vi "Main.vi"() -> ()   [LabVIEW 2017]
doc: "This Continuous Measurement sample project is based on the Queued Message Handler template.\n\nThe Event Handling Loop generates messages based on user interface actions.\n\nThe Message Handling Loop processes messages generated by the Event Handling Loop, or by other messages. There are also Acquisition and Logging message handling loop subVIs, and a chart updating loop."
uses:
  Settings/Settings.ctl
  Acquisition/Hardware Configuration.ctl
  Acquisition/Signal Type.ctl
  Logging/Logging Configuration.ctl
  controls/UI Data.ctl
  controls/UI State.ctl
  support/Message Queue/Enqueue Message (Single).vi
  support/Message Queue/Enqueue Message (Array).vi
  <vilib>/Utility/error.llb/Error Cluster From Error Code.vi
  <vilib>/ErrorRing/Error Ring.xnode
  Acquisition/Acquisition.lvlib
  Logging/Logging.lvlib
  Settings/Settings.lvlib
  support/User Event - Stop/User Event - Stop.lvlib
  support/Message Queue/Message Queue.lvlib
  Settings/Settings Dialog.vi
panel:
  out "Time running":timestamp format="%<%H:%M:%S%1u>T"
  in  "Zero run?":bool
  in  "Start wavemaker":bool
  in  "Preview wave file":bool
  out "Data wave file":waveform(dbl)[](graph)
  in  "Initialize wave maker":bool
  in  "Location wave file":path
  in  "Configure channels":bool
  in  "Exit":bool
  out "Status":string
  in  "Settings":bool
  in  "Stop":bool
  in  "Start":bool
  out "ChannelNames":T1
  out "Offline storage?":bool
  out "Path to offsite data storage":path
  in  "Close and start writing time interval [min]":dbl
  out "Project  code":string
  in  "Zero run testing time [s]":dbl
  in  "Testing time [m]":dbl
  out "Data":waveform(dbl)[](graph)
  # "Flume tank data logging and wave making"
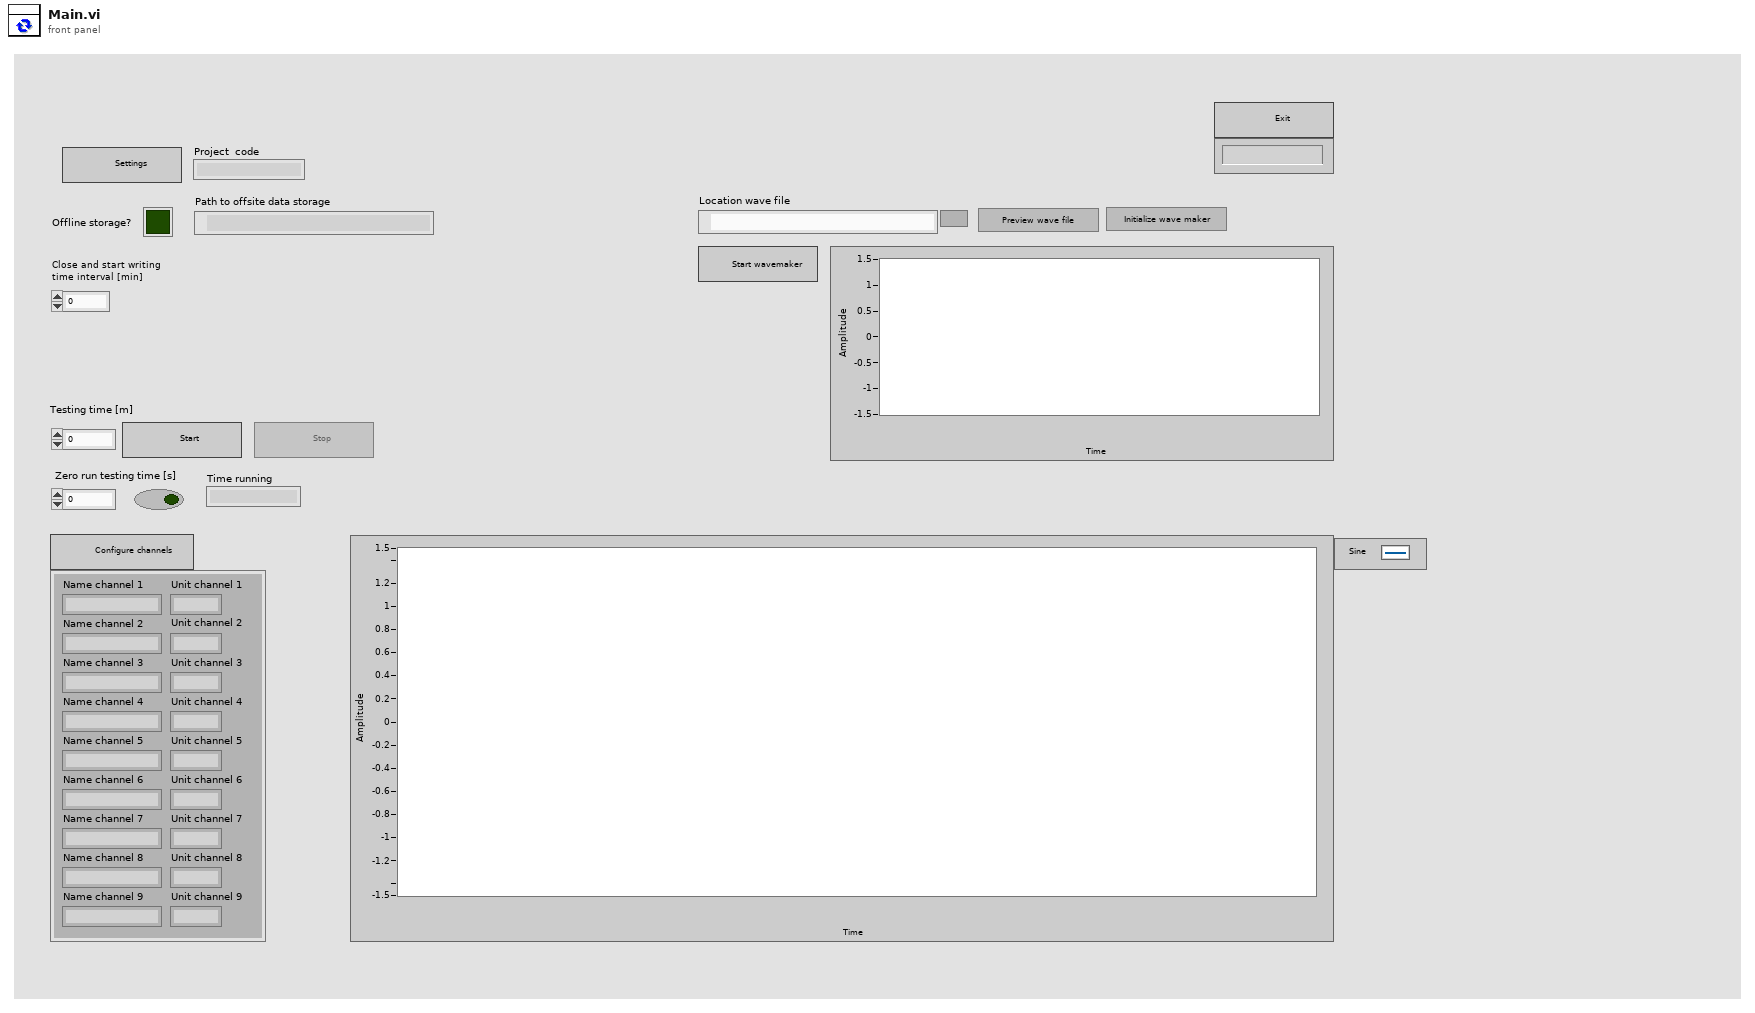
[diagram p1: front panel]
types:
  T1 = cluster{"Name channel 1":string, "Name channel 2":string, "Name channel 3":string, "Name channel 4":string, "Name channel 5":string, "Name channel 6":string, "Name channel 7":string, "Name channel 8":string, "Name channel 9":string, "Unit channel 1":string, "Unit channel 2":string, "Unit channel 3":string, "Unit channel 4":string, "Unit channel 5":string, "Unit channel 6":string, "Unit channel 7":string, "Unit channel 8":string, "Unit channel 9":string}
  T2 = typedef "UI State.ctl" = enum16{"Idle", "Acquiring and Logging", "Waiting for Exit", "Waiting for Exit (Acq Stopped)", "Waiting for Exit (Log Stopped)", "Waiting for Stop", "Waiting for Stop (Acq Stopped)", "Waiting for Stop (Log Stopped)"}
  T3 = typedef "UI Data.ctl" = cluster{"Start Ref":refnum<vi>, "Stop Ref":refnum<vi>, "Settings Ref":refnum<vi>, "Exit Ref":refnum<vi>, "Status Ref":refnum<vi>, "Data Ref":refnum<vi>, "Start wavemaker ref":refnum<vi>, "Preview wave file ref":refnum<vi>, "Config channels ref":refnum<vi>, "Wave preview ref":refnum<vi>}
  T4 = typedef "Settings.lvlib/Settings.ctl" = cluster{"Hardware Configuration":T5, "Logging Configuration":T7, "Project  code":string, "Offline storage?":bool, "Path to offsite data storage":path}
  T5 = typedef "Acquisition.lvlib/Hardware Configuration.ctl" = cluster{"HW Refnum <Replace Me>":string, "Signal Type <Replace Me>":T6}
  T6 = typedef "Acquisition.lvlib/Signal Type.ctl" = enum16{"Sine Wave", "Square with Noise"}
  T7 = typedef "Logging.lvlib/Logging Configuration.ctl" = cluster{"Log File Base Path":path, "TDMS File Reference":refnum<k34>}
  T8 = typedef "Message Queue.lvlib/All Message Queues.ctl" = cluster{"UI":refnum<queue>, "Acquisition":refnum<queue>, "Logging":refnum<queue>}
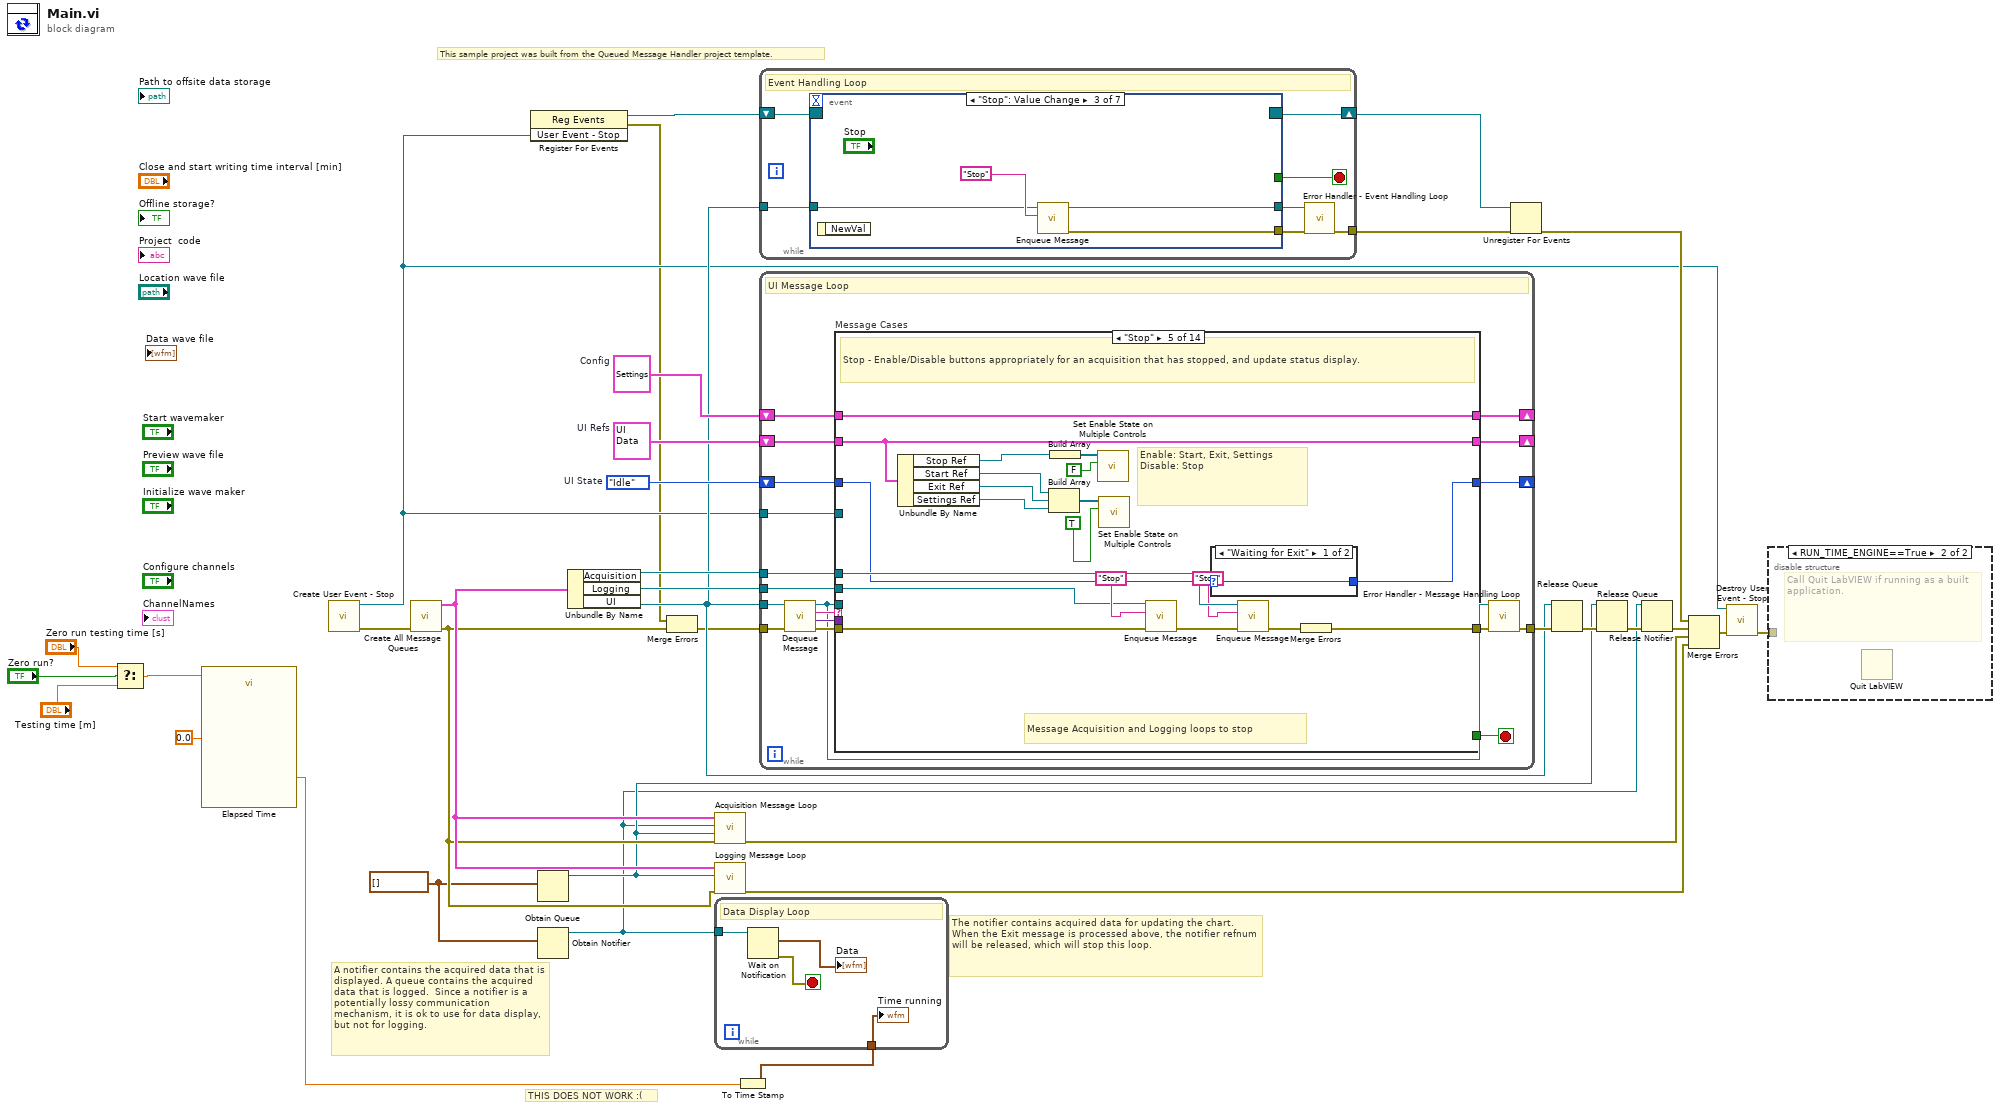
[diagram p0: block diagram]
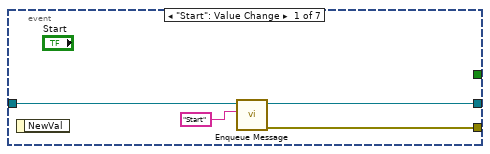
[diagram p3: hidden frame]
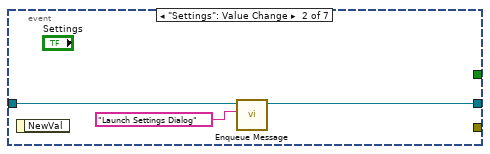
[diagram p4: hidden frame]
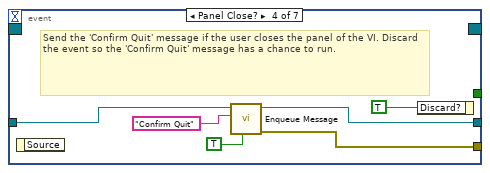
[diagram p5: hidden frame]
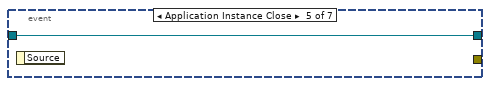
[diagram p6: hidden frame]
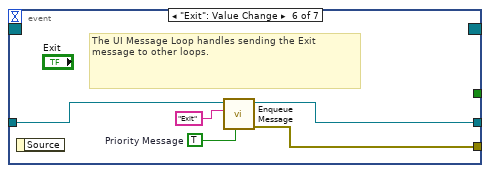
[diagram p7: hidden frame]
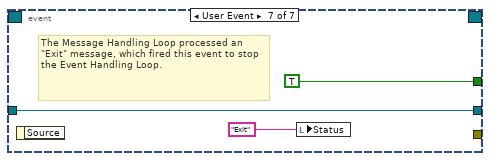
[diagram p8: hidden frame]
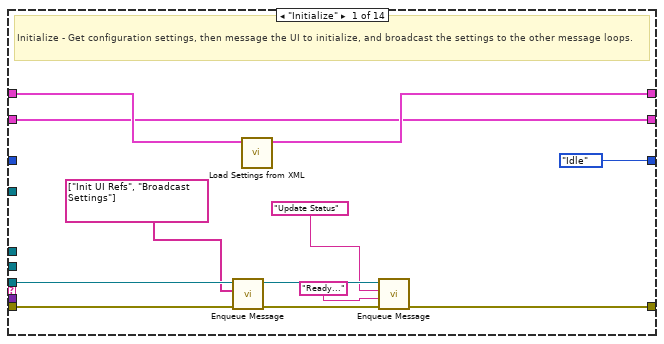
[diagram p9: hidden frame]
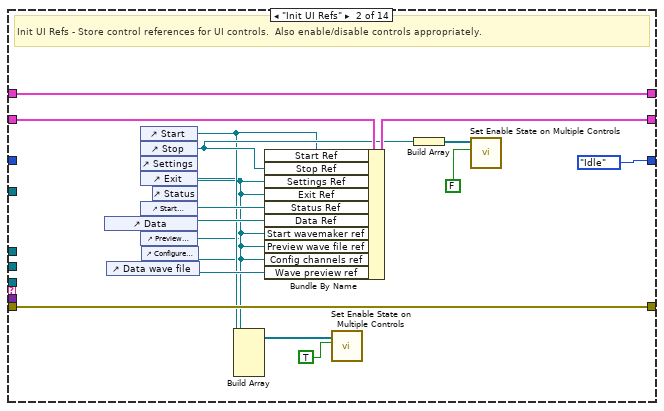
[diagram p10: hidden frame]
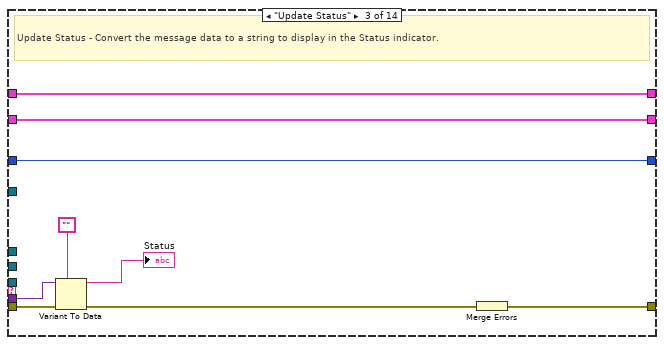
[diagram p11: hidden frame]
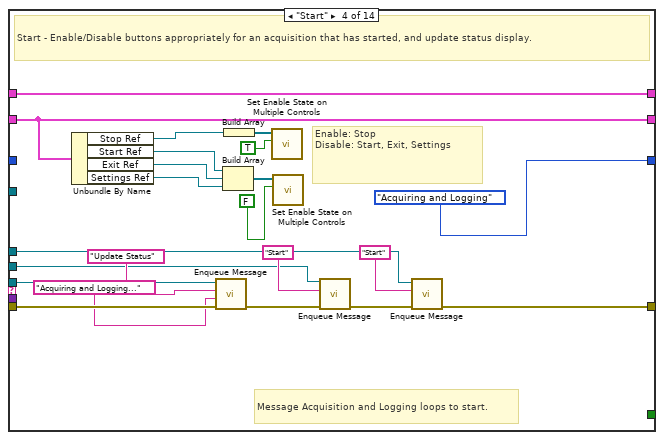
[diagram p12: hidden frame]
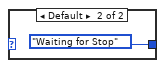
[diagram p13: hidden frame]
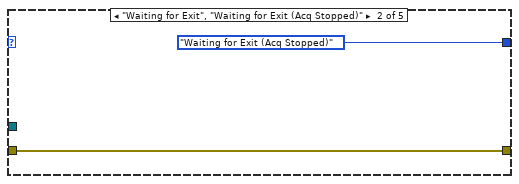
[diagram p15: hidden frame]
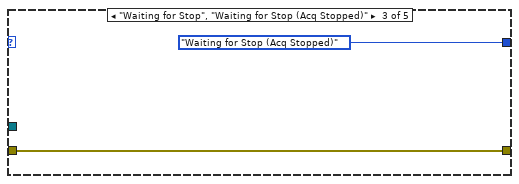
[diagram p16: hidden frame]
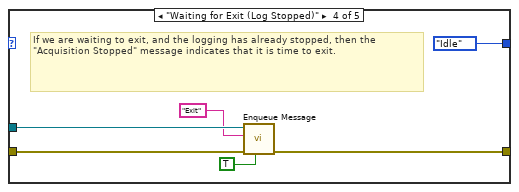
[diagram p17: hidden frame]
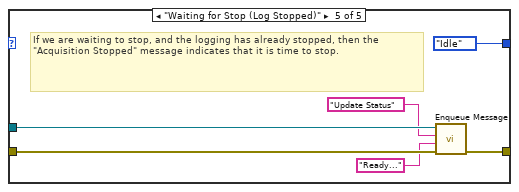
[diagram p18: hidden frame]
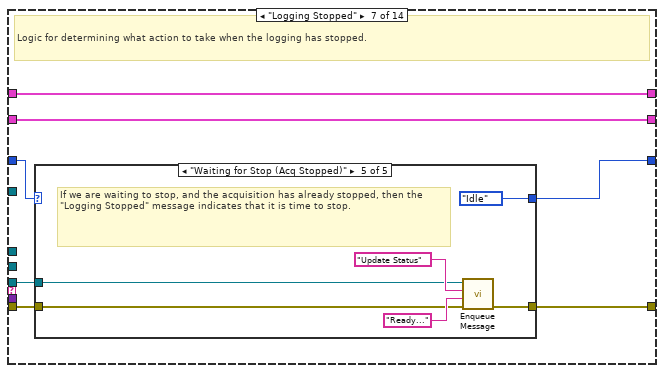
[diagram p19: hidden frame]
diagram:
  w21 = UI_State."Idle"  # UI State
  w12 = waveform(dbl)[] []
  w24 = T3 {"Start Ref"=refnum, "Stop Ref"=refnum, "Settings Ref"=refnum, "Exit Ref"=refnum, "Status Ref"=refnum, "Data Ref"=refnum, "Start wavemaker ref"=refnum, "Preview wave file ref"=refnum, "Config channels ref"=refnum, "Wave preview ref"=refnum}  # UI Refs
  w27 = T4 {"Hardware Configuration"={"HW Refnum <Replace Me>"="", "Signal Type <Replace Me>"=enum."Sine Wave"}, "Logging Configuration"={"Log File Base Path"=path "", "TDMS File Reference"=refnum}, "Project  code"="", "Offline storage?"=FALSE, "Path to offsite data storage"=path ""}  # Config
  # "THIS DOES NOT WORK :("
  # "This sample project was built from the Queued Message Handler project template."
  # "A notifier contains the acquired data that is displayed. A queue contains the acquired data that is logged.  Since a notifier is a potentially lossy communication mechanism, it is ok to use for data display, but not for logging."
  # "The notifier contains acquired data for updating the chart. When the Exit message is processed above, the notifier refnum will be released, which will stop this loop."
  n1 = Select(t="Zero run testing time [s]", s="Zero run?", f="Testing time [m]") -> (s? t:f=w4:dbl)
  n2 = call "Elapsed Time"("Time Target (s)"=w4, "Set Start Time (s)"=0.0) -> ("Elapsed Time (s)"=w1:dbl)  [unwired: 10 in, 7 out]
  n3 = call "Create User Event - Stop.vi"() -> ("error out"=w31:errorcluster, "User Event - Stop"=w10:refnum<user-event>)  [unwired: 10 in]
  n4 = call "Create All Message Queues.vi"("error in (no error)"=w31) -> ("error out"=w28:errorcluster, "Message Queues out"=w30:T8)  [unwired: 9 in]
  n5 = register-events(w10) -> (reference out=w11:refnum<event-registration>, error out=w8:errorcluster)  [unwired: 2 in]
  n6 = Obtain Queue(element data type=w12) -> (queue out=w14:refnum<queue>)  [unwired: 4 in, 2 out]
  n7 = Obtain Notifier(notification data type=w12) -> (notifier out=w13:refnum<notifier>)  [unwired: 3 in, 2 out]
  n8 = Unbundle By Name(w30) -> ("Acquisition"=w23:refnum<queue>, "Logging"=w22:refnum<queue>, "UI"=w19:refnum<queue>)
  n9 = Merge Errors(w8, w28) -> (w9:errorcluster)
  n10 = call "Acquisition Message Loop.vi"("error in (no error)"=w28, "Data Queue"=w14, "Data Notifier"=w13, "Message Queues"=w30) -> ("error out"=w32:errorcluster)  [unwired: 7 in]
  n11 = call "Logging Message Loop.vi"("error in (no error)"=w28, "Data Queue"=w14, "Message Queues"=w30) -> ("error out"=w29:errorcluster)  [unwired: 8 in]
  n12 = To Time Stamp(1:w1) -> (0:w2:timestamp)
  n13 = while "Data Display Loop" {
    tunnel: w13 -> [w38]
    tunnel: w2 -> [w35]
    stop <- w36 stop-if-true
    # "Data Display Loop"
    n14 = Wait on Notification(notifier=w38) -> (notification=→"Data":waveform(dbl)[], error out=w36:errorcluster)  [unwired: 3 in, 2 out]
    "Time running" <- w35
  }
  n15 = while {
    tunnel: w19 -> [w44]
    tunnel: [w41] -> w33
    shift-right: [w43] -> w25
    shift-left: w11 -> [w45]
    stop <- w42 stop-if-true
    # "Event Handling Loop"
    n16 = event shown="[2] \"Stop\": Value Change" {
      selector: w45 -> [_ _ _ _ _ _ _]
      dyn-events: [_ _ _ _ _ _ _] -> w43
      timeout: _ -> [_ _ _ _ _ _ _]
      tunnel: [_ _ _ _ _ _ TRUE ("Discard?")] -> w42
      tunnel: w44 -> [w49 w51 w55 w60 w63 w65 w69]
      tunnel: [w47 _ w54 w58 _ w68 _] -> w40
      tunnel: [w46 w50 w53 w59 w63 w64 w69] -> w39
      event "Start": Value Change {
        n17 = event-data() -> ()  [unwired: 1 in, 1 out]
        n18 = call-poly "Enqueue Message.vi"("Message"="Start", "Message Queue"=w49) -> ("error out"=w47:errorcluster, "dup Message Queue"=w46:refnum<queue>)  [unwired: 8 in]
      }
      event "Settings": Value Change {
        n19 = event-data() -> ()  [unwired: 1 in, 1 out]
        n20 = call-poly "Enqueue Message.vi"("Message"="Launch Settings Dialog", "Message Queue"=w51) -> ("dup Message Queue"=w50:refnum<queue>)  [unwired: 8 in, 1 out]
      }
      event "Stop": Value Change {
        n21 = event-data() -> ()  [unwired: 1 in, 1 out]
        n22 = call-poly "Enqueue Message.vi"("Message"="Stop", "Message Queue"=w55) -> ("error out"=w54:errorcluster, "dup Message Queue"=w53:refnum<queue>)  [unwired: 8 in]
      }
      event Panel Close? {
        # "Send the 'Confirm Quit' message if the user closes the panel of the VI. Discard the event so the 'Confirm Quit' message has a chance to run."
        n23 = event-data() -> ()  [unwired: 1 in, 1 out]
        n24 = call-poly "Enqueue Message.vi"("Priority Message? (F)"=TRUE, "Message"="Confirm Quit", "Message Queue"=w60) -> ("error out"=w58:errorcluster, "dup Message Queue"=w59:refnum<queue>)  [unwired: 7 in]
        n25 = event-data("Discard?"=TRUE) -> ()  [unwired: 1 in, 1 out]
      }
      event Application Instance Close {
        n26 = event-data() -> ()  [unwired: 1 in, 1 out]
      }
      event "Exit": Value Change {
        w66 = TRUE  # Priority Message
        # "The UI Message Loop handles sending the Exit message to other loops."
        n27 = event-data() -> ()  [unwired: 1 in, 1 out]
        n28 = call-poly "Enqueue Message.vi"("Priority Message? (F)"=w66, "Message"="Exit", "Message Queue"=w65) -> ("error out"=w68:errorcluster, "dup Message Queue"=w64:refnum<queue>)  [unwired: 7 in]
      }
      event User Event {
        # "The Message Handling Loop processed an \"Exit\" message, which fired this event to stop the Event Handling Loop."
        n29 = event-data() -> ()  [unwired: 1 in, 1 out]
        n30 = local write "Status"("Exit" ("Exit String")) -> ()
      }
    }
    n31 = call "Error Handler - Event Handling Loop.vi"("error in (no error)"=w40, "Message Queue"=w39) -> ("dup error in"=w41:errorcluster)  [unwired: 8 in, 1 out]
  }
  n32 = while {
    tunnel: w19 -> [w83]
    tunnel: w10 -> [w88]
    shift-right: [w82] -> _
    shift-left: w27 -> [w81]
    shift-right: [w79] -> _
    shift-left: w24 -> [w80]
    tunnel: w23 -> [w78]
    tunnel: w22 -> [w77]
    shift-right: [w72] -> _
    shift-left: w21 -> [w73]
    tunnel: w9 -> [w87]
    tunnel: [w76] -> w34
    stop <- w89 stop-if-true
    # "UI Message Loop"
    n33 = call "Dequeue Message.vi"("error in (no error)"=w87, "Message Queue"=w83) -> ("error out"=w86:errorcluster, "Message Data"=w84:variant, "Message"=w85:string, "dup Message Queue"=w74:refnum<queue>)  [unwired: 6 in]
    n34 = case "Message Cases" shown="\"Stop\"" w85 {
      selector: w85 -> [_ _ _ _ _ _ _ _ _ _ _ _ _ w315]
      tunnel: w74 -> [w93 _ _ w151 _ w176 w201 _ w247 _ w268 _ _ _]
      tunnel: w86 -> [w92 w120 w128 w150 w170 w177 w202 w237 w249 w256 w267 w296 w313 _]
      tunnel: [w97 w120 w129 w133 w171 w174 w199 w241 w242 w259 w266 w306 w312 w314] -> w75
      tunnel: [_ _ _ _ _ _ _ _ _ _ _ TRUE _ _] -> w89
      tunnel: w84 -> [_ _ w127 _ _ _ _ _ _ w260 _ w294 _ _]
      tunnel: w88 -> [_ _ _ _ _ _ _ _ _ _ _ w307 _ _]
      tunnel: [w100 w119 w123 w149 w169 w180 w205 w239 w246 w264 w271 w305 w311 w318] -> w82
      tunnel: w81 -> [w101 w119 w123 w149 w169 w180 w205 w239 w250 w264 w271 w305 w311 w318]
      tunnel: w80 -> [w94 w114 w122 w146 w168 w179 w204 w236 w244 w263 w270 w304 w310 w317]
      tunnel: [w94 w113 w122 w146 w168 w179 w204 w236 w244 w263 w270 w304 w310 w317] -> w79
      tunnel: w78 -> [_ _ _ w132 w155 _ _ w235 _ _ _ w303 _ _]
      tunnel: w77 -> [_ _ _ w135 w158 _ _ w224 _ _ _ w302 _ _]
      tunnel: w73 -> [_ _ w121 _ w152 w178 w203 w234 w243 w258 w269 _ w309 w316]
      tunnel: [UI_State."Idle" ("UI State") UI_State."Idle" ("UI State") w121 UI_State."Acquiring and Logging" ("UI State") w153 w175 w200 w234 w243 w258 w265 UI_State."Idle" ("UI State") w309 w316] -> w72
      frame "Initialize" {
        # "Initialize - Get configuration settings, then message the UI to initialize, and broadcast the settings to the other message loops."
        n35 = call-poly "Enqueue Message.vi"("error in (no error)"=w92, "Message Array"=string[] ["Init UI Refs", "Broadcast Settings"], "Message Queue"=w93) -> ("error out"=w99:errorcluster, "dup Message Queue"=w98:refnum<queue>)  [unwired: 7 in]
        n36 = call "Load Settings from XML.vi"("Settings in"=w101) -> ("Settings out"=w100:T4)  [unwired: 9 in, 1 out]
        n37 = call-poly "Enqueue Message.vi"("error in (no error)"=w99, "Message Data"="Ready..." ("Ready..."), "Message"="Update Status", "Message Queue"=w98) -> ("error out"=w97:errorcluster)  [unwired: 6 in, 1 out]
      }
      frame "Init UI Refs" {
        # "Init UI Refs - Store control references for UI controls.  Also enable/disable controls appropriately."
        n38 = control-ref of="Data"() -> (w110:refnum<vi>)
        n39 = control-ref of="Data wave file"() -> (w109:refnum<vi>)
        n40 = control-ref of="Start"() -> (w108:refnum<vi>)
        n41 = control-ref of="Stop"() -> (w112:refnum<vi>)
        n42 = control-ref of="Settings"() -> (w107:refnum<vi>)
        n43 = control-ref of="Exit"() -> (w106:refnum<vi>)
        n44 = control-ref of="Start wavemaker"() -> (w105:refnum<vi>)
        n45 = control-ref of="Preview wave file"() -> (w104:refnum<vi>)
        n46 = control-ref of="Configure channels"() -> (w103:refnum<vi>)
        n47 = control-ref of="Status"() -> (w111:refnum<vi>)
        n48 = Build Array(w108, w107, w106, w105, w104, w103) -> (w102:refnum<vi>[])
        n49 = Bundle By Name(cluster=w114, "Start Ref"=w108, "Stop Ref"=w112, "Settings Ref"=w107, "Exit Ref"=w106, "Status Ref"=w111, "Data Ref"=w110, "Start wavemaker ref"=w105, "Preview wave file ref"=w104, "Config channels ref"=w103, "Wave preview ref"=w109) -> (w113:T3)
        n50 = call "Set Enable State on Multiple Controls.vi"("Enable?"=TRUE, "Controls"=w102) -> ()  [unwired: 10 in]
        n51 = Build Array(w112) -> (w117:refnum<vi>[])
        n52 = call "Set Enable State on Multiple Controls.vi"("Enable?"=FALSE, "Controls"=w117) -> ()  [unwired: 10 in]
      }
      frame "Update Status" {
        # "Update Status - Convert the message data to a string to display in the Status indicator."
        n53 = Variant To Data(error in=w128, type="", Variant=w127) -> (data=→"Status":string, error out=w125:errorcluster)
        n54 = Merge Errors(w125) -> (w129:errorcluster)
      }
      frame "Start" {
        # "Message Acquisition and Logging loops to start."
        # "Enable: Stop\nDisable: Start, Exit, Settings"
        # "Start - Enable/Disable buttons appropriately for an acquisition that has started, and update status display."
        n55 = Unbundle By Name(w146) -> ("Stop Ref"=w141:refnum<vi>, "Start Ref"=w140:refnum<vi>, "Exit Ref"=w139:refnum<vi>, "Settings Ref"=w138:refnum<vi>)
        n56 = call-poly "Enqueue Message.vi"("error in (no error)"=w150, "Message Data"="Acquiring and Logging..." ("Acquiring and Logging..."), "Message"="Update Status", "Message Queue"=w151) -> ("error out"=w137:errorcluster)  [unwired: 6 in, 1 out]
        n57 = Build Array(w140, w139, w138) -> (w144:refnum<vi>[])
        n58 = Build Array(w141) -> (w143:refnum<vi>[])
        n59 = call "Set Enable State on Multiple Controls.vi"("Enable?"=TRUE, "Controls"=w143) -> ()  [unwired: 10 in]
        n60 = call "Set Enable State on Multiple Controls.vi"("Enable?"=FALSE, "Controls"=w144) -> ()  [unwired: 10 in]
        n61 = call-poly "Enqueue Message.vi"("error in (no error)"=w137, "Message"="Start", "Message Queue"=w135) -> ("error out"=w134:errorcluster)  [unwired: 7 in, 1 out]
        n62 = call-poly "Enqueue Message.vi"("error in (no error)"=w134, "Message"="Start", "Message Queue"=w132) -> ("error out"=w133:errorcluster)  [unwired: 7 in, 1 out]
      }
      frame "Stop" {
        # "Message Acquisition and Logging loops to stop"
        # "Enable: Start, Exit, Settings\nDisable: Stop"
        # "Stop - Enable/Disable buttons appropriately for an acquisition that has stopped, and update status display."
        n63 = Unbundle By Name(w168) -> ("Stop Ref"=w163:refnum<vi>, "Start Ref"=w162:refnum<vi>, "Exit Ref"=w161:refnum<vi>, "Settings Ref"=w160:refnum<vi>)
        n64 = Build Array(w162, w161, w160) -> (w166:refnum<vi>[])
        n65 = Build Array(w163) -> (w165:refnum<vi>[])
        n66 = call "Set Enable State on Multiple Controls.vi"("Enable?"=FALSE, "Controls"=w165) -> ()  [unwired: 10 in]
        n67 = call "Set Enable State on Multiple Controls.vi"("Enable?"=TRUE, "Controls"=w166) -> ()  [unwired: 10 in]
        n68 = call-poly "Enqueue Message.vi"("error in (no error)"=w170, "Message"="Stop", "Message Queue"=w158) -> ("error out"=w157:errorcluster)  [unwired: 7 in, 1 out]
        n69 = case shown="\"Waiting for Exit\"" w152 {
          selector: w152 -> [w172 _]
          tunnel: [w172 UI_State."Waiting for Stop" ("UI State")] -> w153
          frame "Waiting for Exit" {
          }
          frame Default {
          }
        }
        n70 = call-poly "Enqueue Message.vi"("error in (no error)"=w157, "Message"="Stop", "Message Queue"=w155) -> ("error out"=w156:errorcluster)  [unwired: 7 in, 1 out]
        n71 = Merge Errors(w156) -> (w171:errorcluster)
      }
      frame "Acquisition Stopped" {
        # "Logic for determining what action to take when the acquisition has stopped."
        n72 = case shown="Default" w178 {
          selector: w178 -> [w182 _ _ _ _]
          tunnel: w177 -> [w181 w184 w186 w192 w198]
          tunnel: w176 -> [_ _ _ w190 w195]
          tunnel: [w182 UI_State."Waiting for Exit (Acq Stopped)" ("UI State") UI_State."Waiting for Stop (Acq Stopped)" ("UI State") UI_State."Idle" ("UI State") UI_State."Idle" ("UI State")] -> w175
          tunnel: [w181 w184 w186 w191 w196] -> w174
          frame Default {
          }
          frame "Waiting for Exit", "Waiting for Exit (Acq Stopped)" {
          }
          frame "Waiting for Stop", "Waiting for Stop (Acq Stopped)" {
          }
          frame "Waiting for Exit (Log Stopped)" {
            # "If we are waiting to exit, and the logging has already stopped, then the \"Acquisition Stopped\" message indicates that it is time to exit."
            n73 = call-poly "Enqueue Message.vi"("Priority Message? (F)"=TRUE, "error in (no error)"=w192, "Message"="Exit", "Message Queue"=w190) -> ("error out"=w191:errorcluster)  [unwired: 6 in, 1 out]
          }
          frame "Waiting for Stop (Log Stopped)" {
            # "If we are waiting to stop, and the logging has already stopped, then the \"Acquisition Stopped\" message indicates that it is time to stop."
            n74 = call-poly "Enqueue Message.vi"("error in (no error)"=w198, "Message Data"="Ready..." ("Ready..."), "Message"="Update Status", "Message Queue"=w195) -> ("error out"=w196:errorcluster)  [unwired: 6 in, 1 out]
          }
        }
      }
      frame "Logging Stopped" {
        # "Logic for determining what action to take when the logging has stopped."
        n75 = case shown="\"Waiting for Stop (Acq Stopped)\"" w203 {
          selector: w203 -> [w207 _ _ _ _]
          tunnel: w202 -> [w206 w209 w211 w217 w220]
          tunnel: w201 -> [_ _ _ w215 w219]
          tunnel: [w207 UI_State."Waiting for Exit (Log Stopped)" ("UI State") UI_State."Waiting for Stop (Log Stopped)" ("UI State") UI_State."Idle" ("UI State") UI_State."Idle" ("UI State")] -> w200
          tunnel: [w206 w209 w211 w216 w218] -> w199
          frame Default {
          }
          frame "Waiting for Exit", "Waiting for Exit (Log Stopped)" {
          }
          frame "Waiting for Stop", "Waiting for Stop (Log Stopped)" {
          }
          frame "Waiting for Exit (Acq Stopped)" {
            # "If we are waiting to exit, and the acquisition has already stopped, then the \"Logging Stopped\" message indicates that it is time to exit."
            n76 = call-poly "Enqueue Message.vi"("Priority Message? (F)"=TRUE, "error in (no error)"=w217, "Message"="Exit", "Message Queue"=w215) -> ("error out"=w216:errorcluster)  [unwired: 6 in, 1 out]
          }
          frame "Waiting for Stop (Acq Stopped)" {
            # "If we are waiting to stop, and the acquisition has already stopped, then the \"Logging Stopped\" message indicates that it is time to stop."
            n77 = call-poly "Enqueue Message.vi"("error in (no error)"=w220, "Message Data"="Ready..." ("Ready..."), "Message"="Update Status", "Message Queue"=w219) -> ("error out"=w218:errorcluster)  [unwired: 6 in, 1 out]
          }
        }
      }
      frame "Broadcast settings" {
        w228 = "Update Settings" ("Message")
        # "Broadcast settings - Send the 'Update Settings' message to the Logging and Acquisition message loops."
        n78 = Unbundle By Name(w239) -> ("Hardware Configuration"=w238:T5, "Logging Configuration"=w233:T7, "Project  code"=w227:string, "Offline storage?"=w226:bool, "Path to offsite data storage"=w225:path)
        n79 = call-poly "Enqueue Message.vi"("Message Data"=w238, "Message"=w228, "Message Queue"=w235) -> ("error out"=w240:errorcluster)  [unwired: 7 in, 1 out]
        n80 = call-poly "Enqueue Message.vi"("error in (no error)"=w240, "Message Data"=w233, "Message"=w228, "Message Queue"=w224) -> ("error out"=w232:errorcluster)  [unwired: 6 in, 1 out]
        n81 = call-poly "Enqueue Message.vi"("error in (no error)"=w232, "Message Data"=w227, "Message"=w228, "Message Queue"=w224) -> ("error out"=w231:errorcluster)  [unwired: 6 in, 1 out]
        n82 = call-poly "Enqueue Message.vi"("error in (no error)"=w231, "Message Data"=w226, "Message"=w228, "Message Queue"=w224) -> ("error out"=w230:errorcluster)  [unwired: 6 in, 1 out]
        n83 = call-poly "Enqueue Message.vi"("error in (no error)"=w230, "Message Data"=w225, "Message"=w228, "Message Queue"=w224) -> ("error out"=w229:errorcluster)  [unwired: 6 in, 1 out]
        n84 = Merge Errors(w229, w237) -> (w241:errorcluster)
      }
      frame "Launch Settings Dialog" {
        # "Launch Settings Dialog - Launch the Settings Dialog when the user clicks the 'Settings' button."
        n85 = call-by-ref "?"("error in (no error)"=w249, "Settings in"=w250) -> ("error out"=w245:errorcluster, "Cancelled?"=w248:bool, "Settings out"=w246:T4)  [unwired: 8 in, 3 out]
        n86 = case shown="False" w248 {
          tunnel: w247 -> [w254 _]
          tunnel: w245 -> [w253 w255]
          tunnel: [w252 w255] -> w242
          frame False {
            n87 = call-poly "Enqueue Message.vi"("error in (no error)"=w253, "Message"="Broadcast Settings", "Message Queue"=w254) -> ("error out"=w252:errorcluster)  [unwired: 7 in, 1 out]
          }
          frame True {
          }
        }
      }
      frame "Error" {
        # "Error - Display an error dialog. This message is sent by the \"Error Handler\" VIs at the end of other loops in this application."
        n88 = Variant To Data(error in=w256, type=errorcluster {"status"=FALSE, "code"=0, "source"=""} ("error constant"), Variant=w260) -> (data=w257:errorcluster, error out=w261:errorcluster)
        n89 = call <vilib>:"Simple Error Handler.vi"("error in (no error)"=w257) -> ()  [unwired: 4 in, 5 out]
        n90 = Merge Errors(w261) -> (w259:errorcluster)
      }
      frame "Confirm Quit" {
        # "Confirm Quit - Message that can confirm whether or not the user wants to exit the application."
        n91 = case shown="Default" w269 {
          tunnel: w268 -> [w277 w281]
          tunnel: w267 -> [w276 w280]
          tunnel: [w275 w279] -> w266
          tunnel: [UI_State."Idle" ("UI State") w278] -> w265
          frame Default {
            # "If 'Confirm Quit' comes in while the system is idle, there is no need for a confirmation message."
            n92 = call-poly "Enqueue Message.vi"("Priority Message? (F)"=TRUE, "error in (no error)"=w276, "Message"="Exit", "Message Queue"=w277) -> ("error out"=w275:errorcluster)  [unwired: 6 in, 1 out]
          }
          frame "Acquiring and Logging" {
            n93 = Two Button Dialog(message="Are you sure you want to quit while the acquisition is running?" ("Confirm Quit Message"), 1:"No" ("No"), 2:"Yes" ("Yes")) -> (T button?=w282:bool)
            n94 = case shown="True" w282 {
              tunnel: w281 -> [_ w291]
              tunnel: w280 -> [w287 w292]
              tunnel: [w287 w290] -> w279
              tunnel: [UI_State."Acquiring and Logging" ("UI State") UI_State."Waiting for Exit" ("UI State")] -> w278
              frame False {
                # "User did not want to quit."
              }
              frame True {
                n95 = call-poly "Enqueue Message.vi"("error in (no error)"=w292, "Message"="Stop", "Message Queue"=w291) -> ("error out"=w290:errorcluster)  [unwired: 7 in, 1 out]
              }
            }
          }
        }
      }
      frame "Exit" {
        w298 = TRUE ("Priority Message? (F)")
        w299 = "Exit" ("Message")
        # "Popup an error dialog if 'Exit' was called as a result of an error."
        # "Stop the VI"
        # "Exit - Send Exit messages to the Acquisition and Logging loops, and fire the user event to stop the Event Handling Loop."
        n96 = Variant To Data(type=errorcluster {"status"=FALSE, "code"=0, "source"=""} ("error constant"), Variant=w294) -> (data=w293:errorcluster)  [unwired: 1 in, 1 out]
        n97 = call <vilib>:"Simple Error Handler.vi"("error in (no error)"=w293) -> ()  [unwired: 4 in, 5 out]
        n98 = call-poly "Enqueue Message.vi"("Priority Message? (F)"=w298, "error in (no error)"=w296, "Message"=w299, "Message Queue"=w303) -> ("error out"=w300:errorcluster)  [unwired: 6 in, 1 out]
        n99 = call-poly "Enqueue Message.vi"("Priority Message? (F)"=w298, "error in (no error)"=w300, "Message"=w299, "Message Queue"=w302) -> ("error out"=w297:errorcluster)  [unwired: 6 in, 1 out]
        n100 = call "Fire User Event - Stop.vi"("error in (no error)"=w297, "User Event - Stop"=w307) -> ("error out"=w306:errorcluster)  [unwired: 9 in]
      }
      frame "---Copy This Frame---" {
        # "Duplicate this frame when creating new messages.  Change this comment in the duplicated frame to describe this message."
        n101 = Merge Errors(w313) -> (w312:errorcluster)
      }
      frame Default {
        # "'Default' case only runs if there is a message that isn't defined in any of the other cases.  Output a programming error."
        n102 = xnode "Error Ring"("parameter 0"=w315) -> ("error out"=w314:errorcluster)
      }
    }
    n103 = call "Error Handler - Message Handling Loop.vi"("error in (no error)"=w75, "Message Queue"=w74) -> ("dup error in"=w76:errorcluster)  [unwired: 8 in, 1 out]
  }
  n104 = Unregister For Events(event registration refnum=w25, error in=w33) -> (error out=w26:errorcluster)
  n105 = Release Queue(queue=w19, error in (no error)=w34) -> (error out=w17:errorcluster)  [unwired: 1 in, 2 out]
  n106 = Release Queue(queue=w14, error in (no error)=w17) -> (error out=w16:errorcluster)  [unwired: 1 in, 2 out]
  n107 = Release Notifier(notifier=w13, error in (no error)=w16) -> (error out=w15:errorcluster)  [unwired: 1 in, 2 out]
  n108 = Merge Errors(w26, w15, w32, w29) -> (w20:errorcluster)
  n109 = call "Destroy User Event - Stop.vi"("error in (no error)"=w20, "User Event - Stop"=w10) -> ("error out"=w18:errorcluster)  [unwired: 9 in]
  n110 = disable-structure shown="RUN_TIME_ENGINE==True" {
    disable-tunnel: w18 -> [_ _]
    frame condition #0 (active) {
    }
    frame condition #1 {
      # "Call Quit LabVIEW if running as a built application."
      n111 = Quit LabVIEW() -> ()  [unwired: 1 in]
    }
  }
